vi "init.vi"(8 "error in (no error)":errorcluster, 10 "inputs":u16[][](array[numeric]), 11 "MeasurementResult in":refnum<class "MeasurementResult.lvclass">) -> (0 "error out":errorcluster, 3 "MeasurementResult out":refnum<class "MeasurementResult.lvclass">)   [LabVIEW 2017, in "MeasurementResult.lvclass"]
doc: "Create a new MeasurementResult object"
uses:
  MeasurementResult.lvclass
  MeasurementResult.lvclass/MeasurementResult.ctl
panel:
  # "2d array of u16"
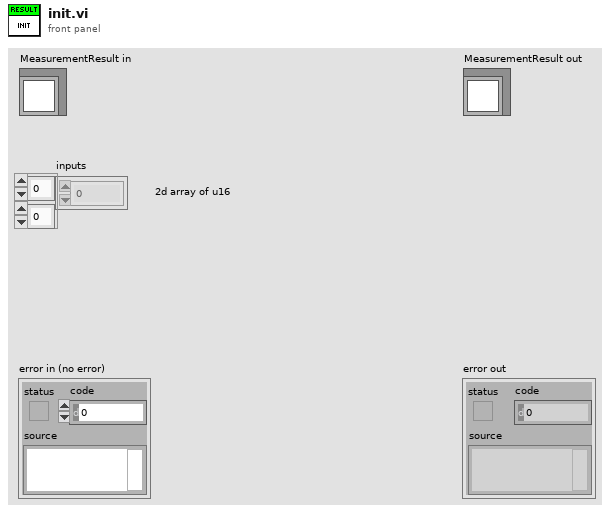
[diagram p1: front panel]
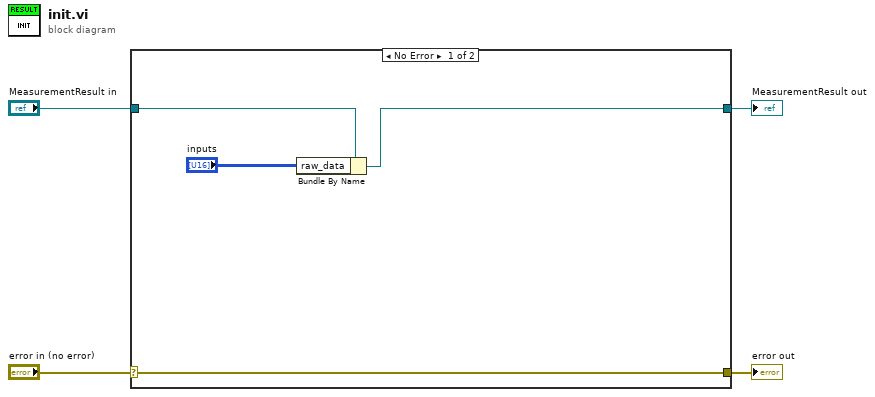
[diagram p0: block diagram]
diagram:
  n1 = case shown="No Error" "error in (no error)" {
    selector: "error in (no error)" -> [w8 w10]
    tunnel: [w8 w10] -> w3
    tunnel: [w6 w9] -> w1
    tunnel: "MeasurementResult in" -> [w7 w9]
    frame No Error {
      n2 = Bundle By Name(cluster=w7, "raw_data"="inputs") -> (w6:refnum<class "MeasurementResult.lvclass">)
    }
    frame Error {
    }
  }
  "error out" <- w3
  "MeasurementResult out" <- w1
